vi "Log Message FGV.vi"(7 "FGV Cmd":T1(ring), 8 "error in (no error)":errorcluster, 9 "Error In":errorcluster, 10 "Message In":string) -> (0 "error out":errorcluster)   [LabVIEW 2016, in "PXImc Custom Device Engine.lvlib"]
uses:
  Engine/PXImc Custom Device Engine.lvlib
  <vilib>/NI VeriStand/Custom Device Tools/Custom Device Utility Library/Custom Device Utility Library.lvlib
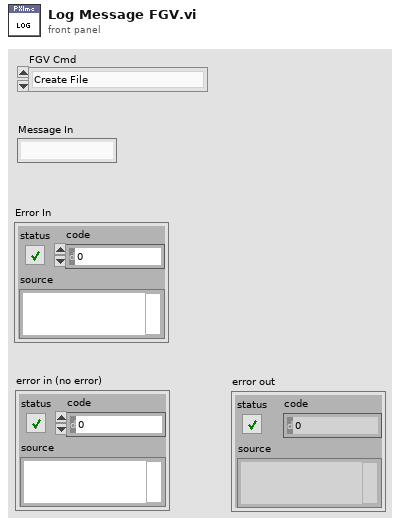
[diagram p1: front panel]
types:
  T1 = enum16{"Create File", "Log Message", "Log Error", "Log TimeStamp", "Close File"}
  T2 = enum16{"open", "replace", "create", "open or create", "replace or create", "replace or create with confirmation"}
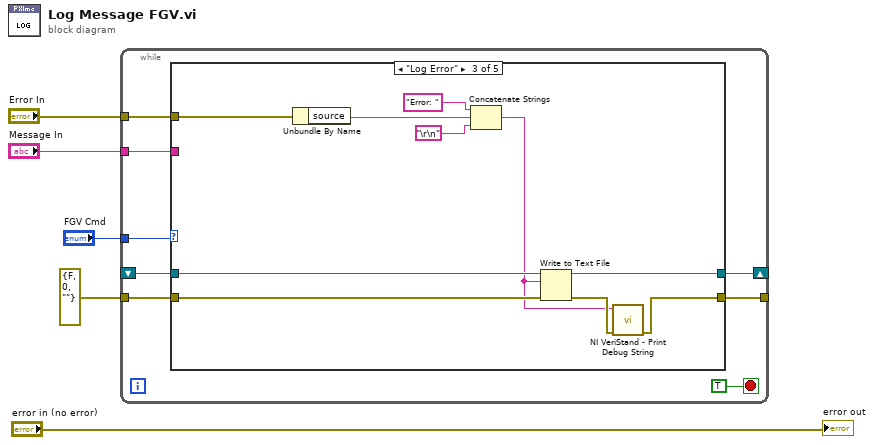
[diagram p0: block diagram]
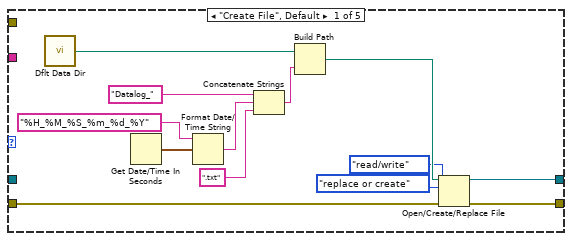
[diagram p2: hidden frame]
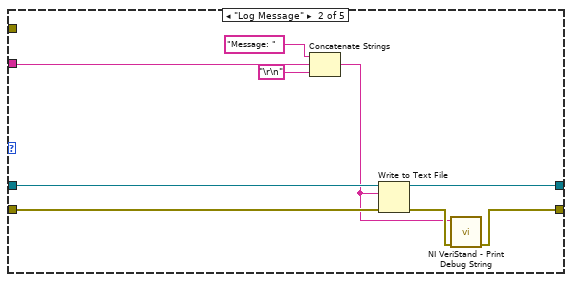
[diagram p3: hidden frame]
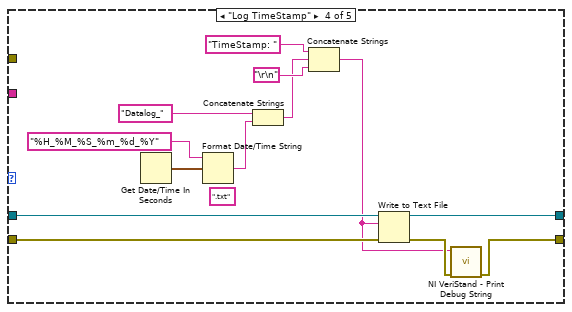
[diagram p4: hidden frame]
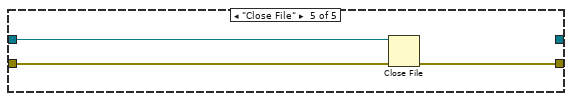
[diagram p5: hidden frame]
diagram:
  n1 = while {
    tunnel: "FGV Cmd" -> [w13]
    tunnel: errorcluster {"status"=FALSE, "code"=0, "source"=""} ("error constant") -> [w12]
    tunnel: [w11] -> _
    shift-right: [w9] -> _
    shift-left: _ -> [w8]
    tunnel: "Error In" -> [w7]
    tunnel: "Message In" -> [w6]
    stop <- TRUE stop-if-true
    n2 = case shown="\"Log Error\"" w13 {
      tunnel: w12 -> [w23 w34 w44 w57 w60]
      tunnel: [w22 w31 w41 w54 w59] -> w11
      tunnel: [w21 w33 w43 w56 _] -> w9
      tunnel: w8 -> [_ w35 w45 w58 w61]
      tunnel: w7 -> [_ _ w37 _ _]
      tunnel: w6 -> [_ w28 _ _ _]
      frame "Create File", Default {
        n3 = call <vilib>:"Dflt Data Dir.vi"() -> ("App:Default Data Directory"=w26:path)
        n4 = Get Date/Time In Seconds() -> (seconds since 1Jan1904=w18:timestamp)
        n5 = Format Date/Time String(time format string (%c)="%H_%M_%S_%m_%d_%Y", seconds (now)=w18) -> (date/time string=w16:string)  [unwired: 1 in]
        n6 = Concatenate Strings("Datalog_" ("name or relative path"), w16, ".txt" ("string")) -> (w14:string)
        n7 = Build Path(base path=w26, name or relative path=w14) -> (appended path=w25:path)
        n8 = Open/Create/Replace File(file path (use dialog)=w25, error in=w23, operation (0:open)=T2."replace or create", access (0:read/write)=enum16{"read/write", "read-only", "write-only"}."read/write") -> (refnum out=w21:refnum<file>, error out=w22:errorcluster)  [unwired: 2 in, 1 out]
      }
      frame "Log Message" {
        n9 = Concatenate Strings("Message: " ("string"), w28, "\r\n") -> (w27:string)
        n10 = Write to Text File(file (use dialog)=w35, text=w27, error in=w34) -> (refnum out=w33:refnum<file>, error out=w32:errorcluster)  [unwired: 1 in, 1 out]
        n11 = call <vilib>:"NI VeriStand - Print Debug String.vi"("error in (no error)"=w32, "Message"=w27) -> ("error out"=w31:errorcluster)  [unwired: 9 in]
      }
      frame "Log Error" {
        n12 = Unbundle By Name(w37) -> ("source"=w40:string)
        n13 = Concatenate Strings("Error: " ("string"), w40, "\r\n") -> (w36:string)
        n14 = Write to Text File(file (use dialog)=w45, text=w36, error in=w44) -> (refnum out=w43:refnum<file>, error out=w42:errorcluster)  [unwired: 1 in, 1 out]
        n15 = call <vilib>:"NI VeriStand - Print Debug String.vi"("error in (no error)"=w42, "Message"=w36) -> ("error out"=w41:errorcluster)  [unwired: 9 in]
      }
      frame "Log TimeStamp" {
        (unwired) ".txt" ("string")
        n16 = Get Date/Time In Seconds() -> (seconds since 1Jan1904=w49:timestamp)
        n17 = Format Date/Time String(time format string (%c)="%H_%M_%S_%m_%d_%Y", seconds (now)=w49) -> (date/time string=w47:string)  [unwired: 1 in]
        n18 = Concatenate Strings("Datalog_" ("name or relative path"), w47) -> (w46:string)
        n19 = Concatenate Strings("TimeStamp: " ("string"), w46, "\r\n") -> (w51:string)
        n20 = Write to Text File(file (use dialog)=w58, text=w51, error in=w57) -> (refnum out=w56:refnum<file>, error out=w55:errorcluster)  [unwired: 1 in, 1 out]
        n21 = call <vilib>:"NI VeriStand - Print Debug String.vi"("error in (no error)"=w55, "Message"=w51) -> ("error out"=w54:errorcluster)  [unwired: 9 in]
      }
      frame "Close File" {
        n22 = Close File(refnum=w61, error in=w60) -> (error out=w59:errorcluster)  [unwired: 1 out]
      }
    }
  }
  "error out" <- "error in (no error)"
